vi "Audio ACQ & Store.vi"() -> ()   [LabVIEW 2020]
uses:
  support/typedefs/Record_States.ctl
  <vilib>/sound2/lvsound2.llb/Sound Input Task ID.ctl
  <vilib>/event_ctls.llb/usereventprio.ctl
  <vilib>/sound2/lvsound2.llb/Sampling Mode.ctl
  support/typedefs/Audio_Data.ctl
  <vilib>/sound2/lvsound2.llb/Sound Data Format.ctl
  <vilib>/sound2/lvsound2.llb/Sound Input Read (DBL).vi
panel:
  out "Audio":waveform(dbl)[](graph)
  in  "Refresh List":bool
  in  "Plot Selection":T1(array[cluster])
  in  "Audio Settings":T2={"Microphone Input Device"=0, "Channels"=1, "Audio Depth"=1, "Sampling Frequncy Hz"=44100.0} {"Sampling Frequncy Hz" items=["11025"=11025.0, "22050"=22050.0, "44100"=44100.0]; "Audio Depth" items=["8", "16"]; "Channels" items=["1", "2"]; "Microphone Input Device" items=["Microphone (USB 2.0 Camera)", "Microphone (2- High Definition Audio Device)", "Microphone (2- High Definition Audio Device)"]}
  in  "Clear":bool
  in  "Pause/Resume":bool
  in  "Stop":bool
  in  "Save":bool
  in  "Record":bool
  in  "Storage Path":path
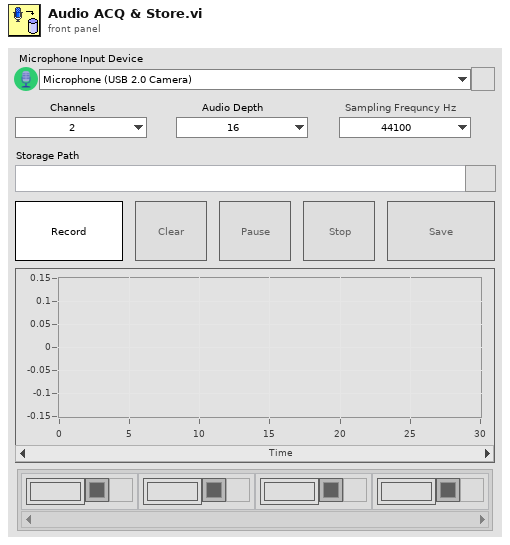
[diagram p1: front panel]
types:
  T1 = cluster{"Plot Name":string, "Plot Color":u32, "Visibility":bool}[]
  T2 = cluster{"Microphone Input Device":u32, "Channels":i32, "Audio Depth":i32, "Sampling Frequncy Hz":dbl}
  T3 = typedef "Record_States.ctl" = enum16{"Initialize", "Load Device List", "Load Device Info", "Respond UI", "Record", "Start ACQ", "Update Plot Propts", "Select Plots", "Clear", "Pause", "Resume", "Stop", "Save", "Exit"}
  T4 = typedef "Sound Input Task ID.ctl" = u32
  T5 = cluster{"channels":i32[], "depths":i32[], "minFreq":dbl, "maxFreq":dbl}[]
  T6 = enum8{"Enabled", "Disabled", "Disabled and Grayed Out"}
  T7 = cluster{"channels":i32[], "depths":i32[], "minFreq":dbl, "maxFreq":dbl}
  T8 = typedef "Audio_Data.ctl" = cluster{"Device":u32, "sound format":T9, "data":refnum<user-event>, "Pause?":bool}
  T9 = typedef "Sound Data Format.ctl" = cluster{"sample rate (S/s)":dbl, "number of channels":i32, "bits per sample":i32}
  T10 = typedef "usereventprio.ctl" = enum32{"high priority", "normal priority"}
  T11 = typedef "Sampling Mode.ctl" = i32
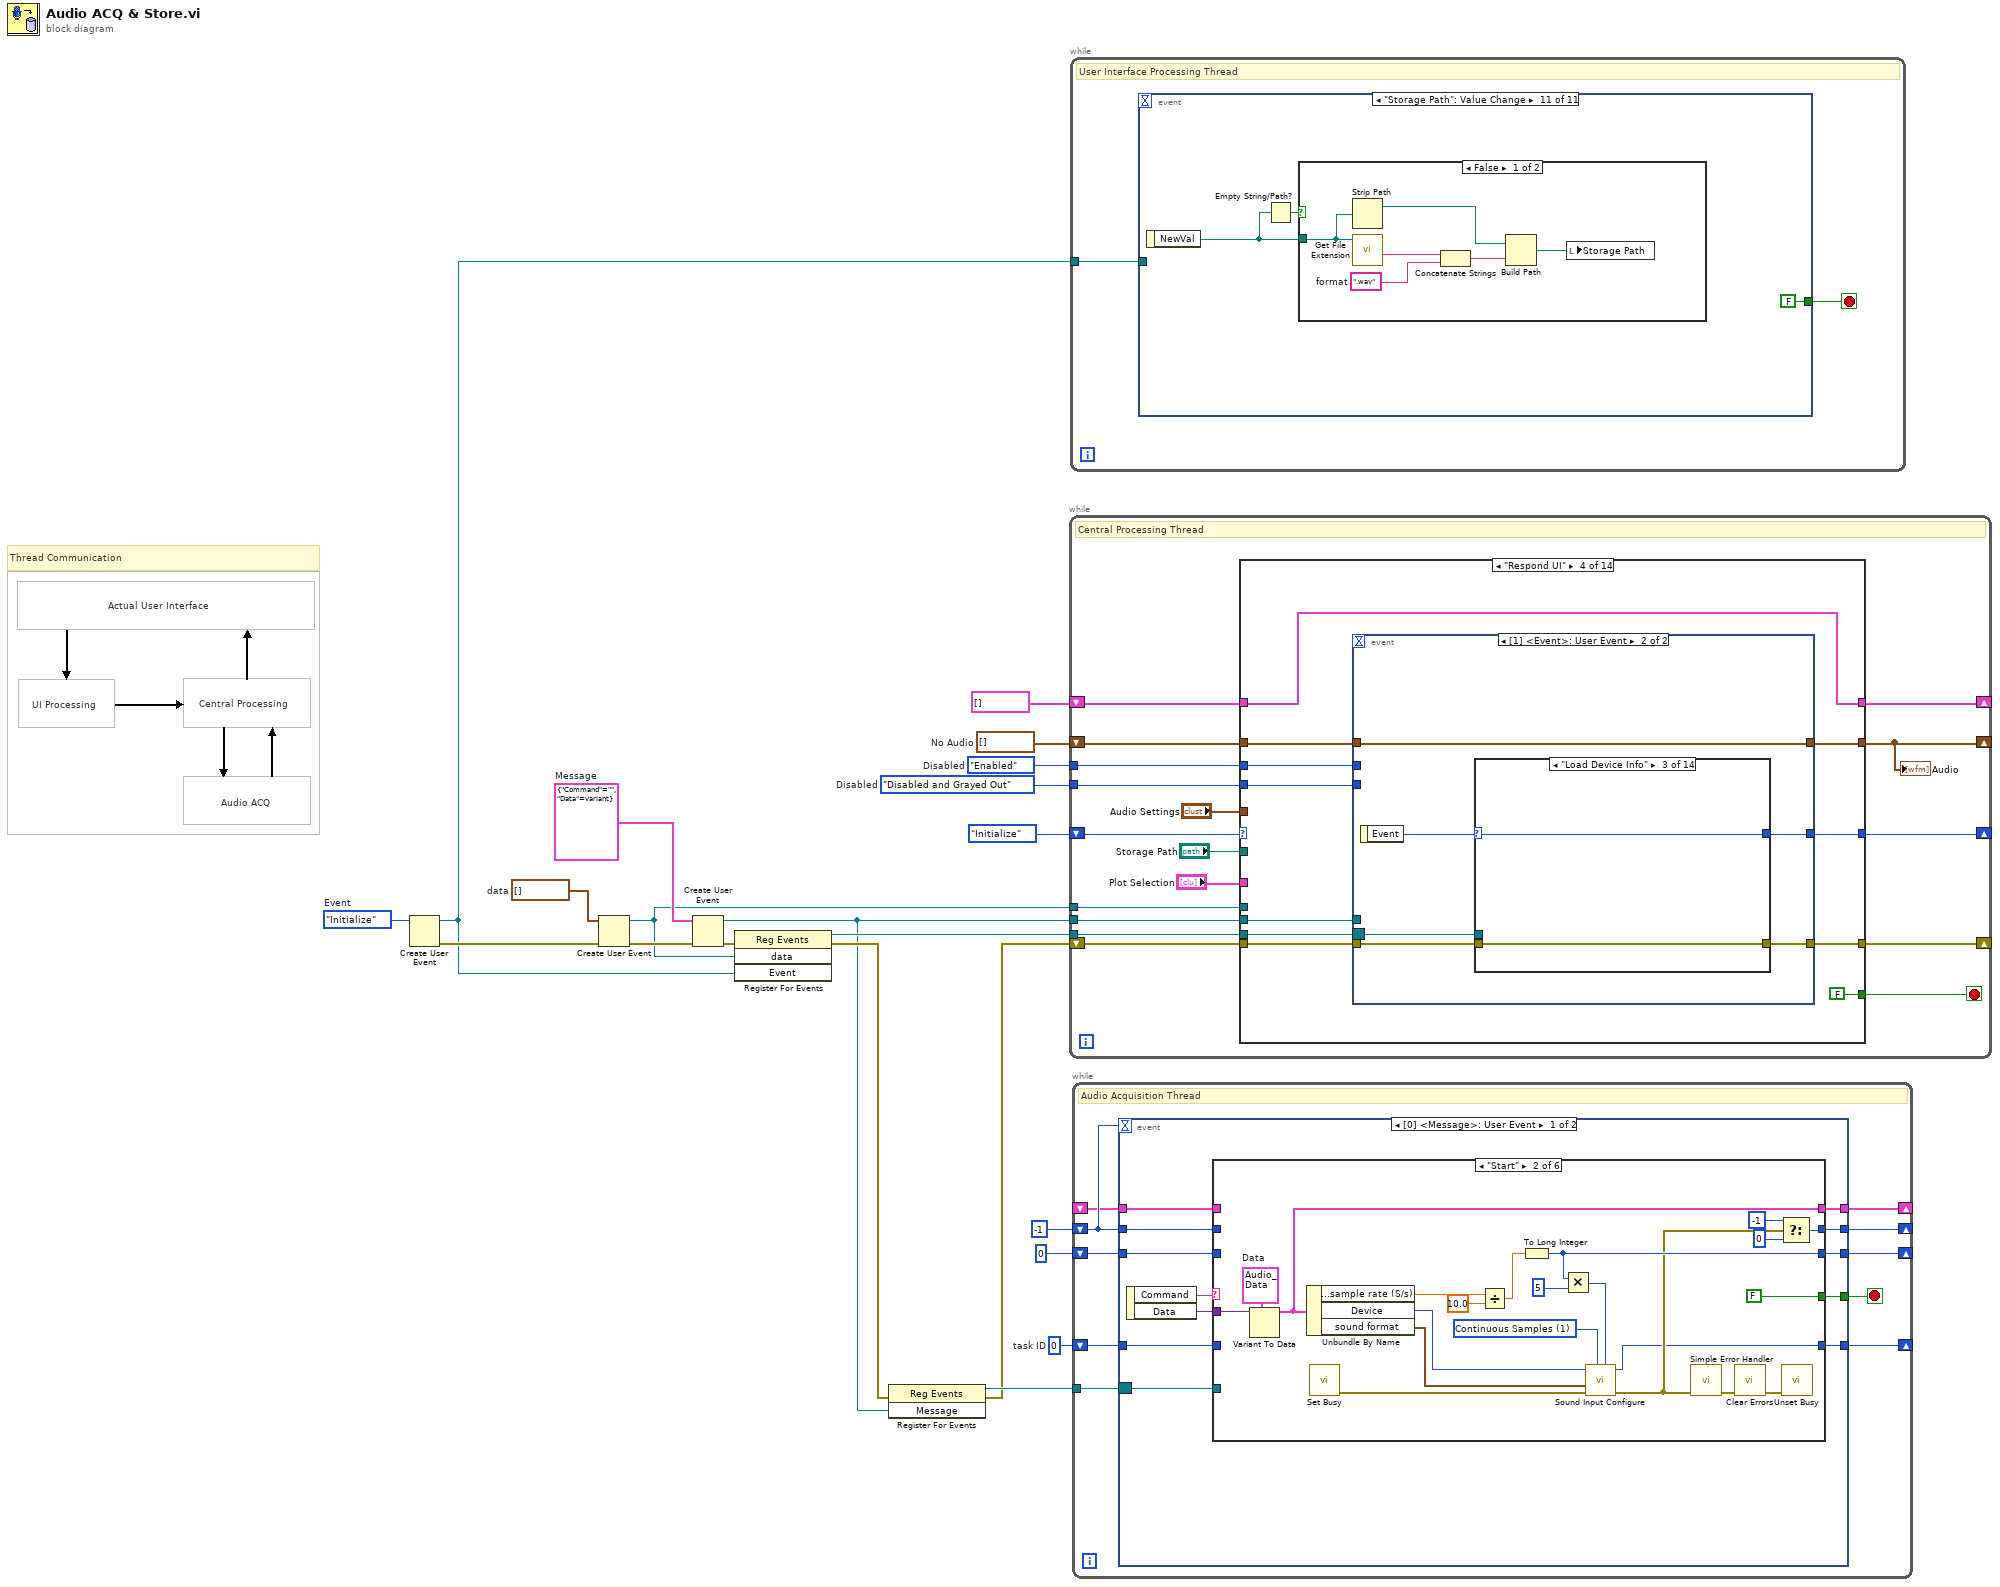
[diagram p0: block diagram]
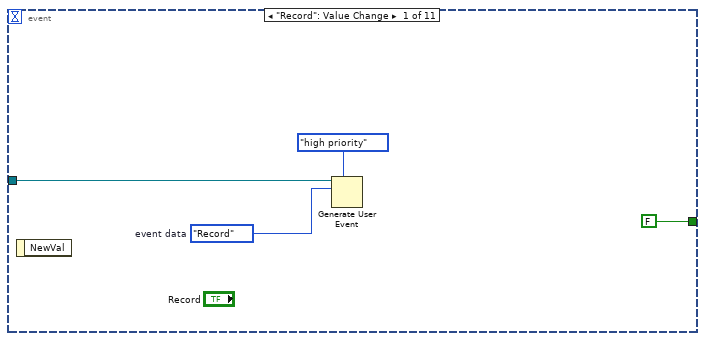
[diagram p2: hidden frame]
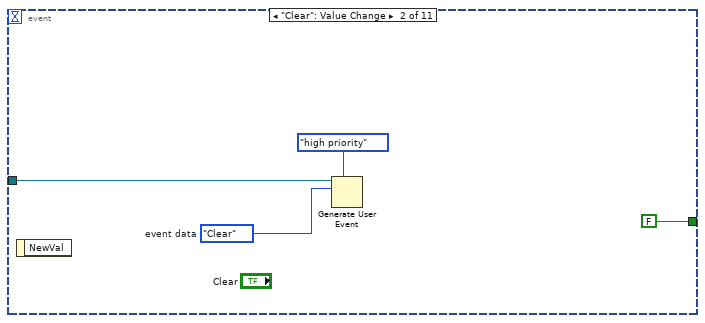
[diagram p3: hidden frame]
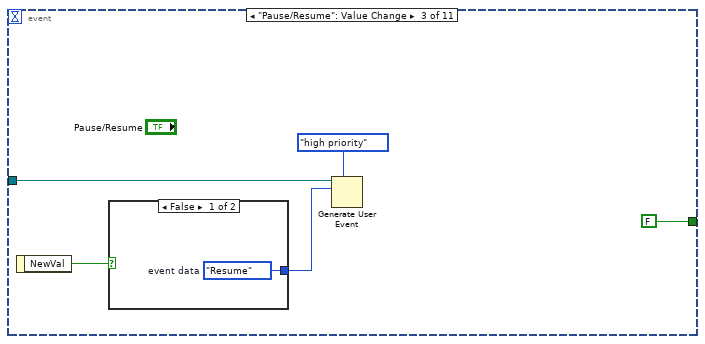
[diagram p4: hidden frame]
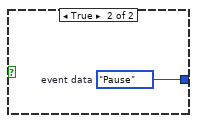
[diagram p5: hidden frame]
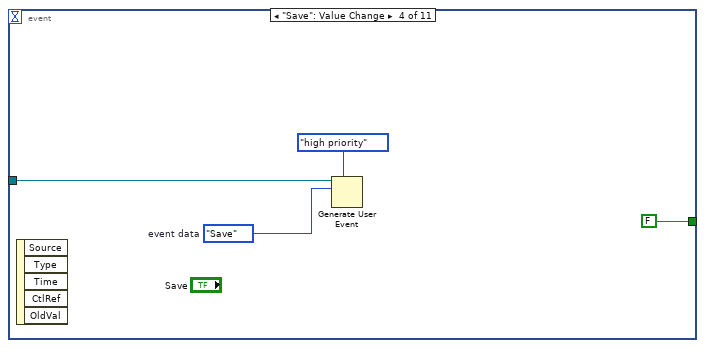
[diagram p6: hidden frame]
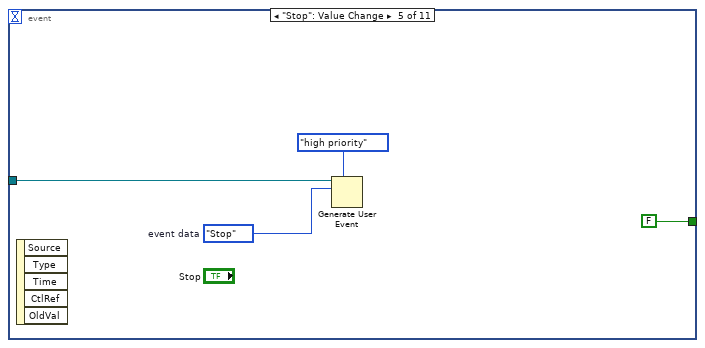
[diagram p7: hidden frame]
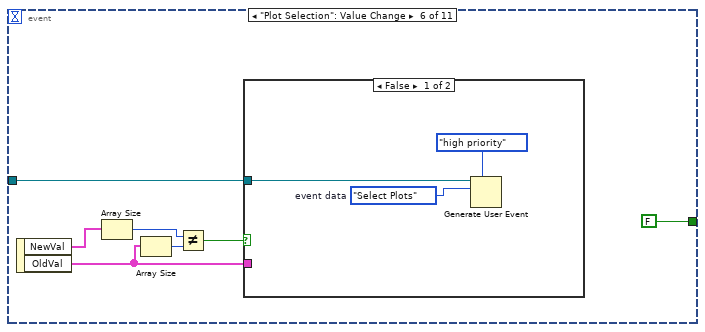
[diagram p8: hidden frame]
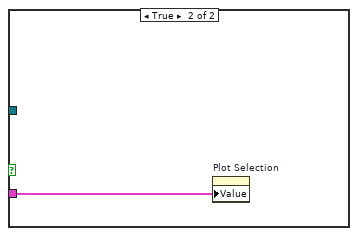
[diagram p9: hidden frame]
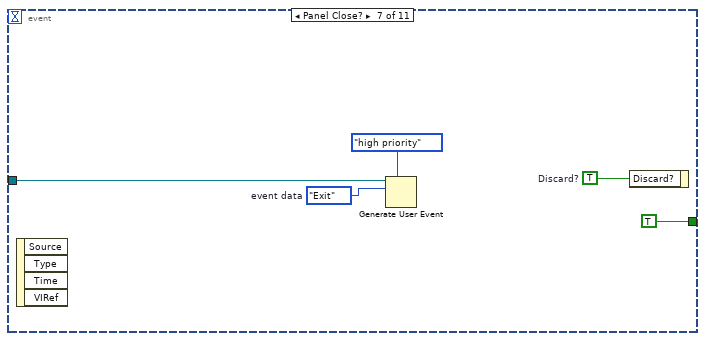
[diagram p10: hidden frame]
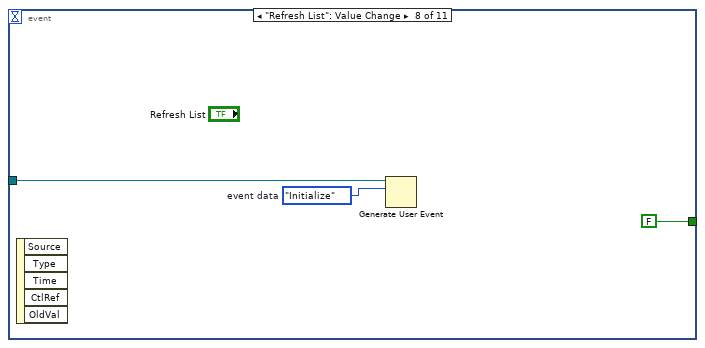
[diagram p11: hidden frame]
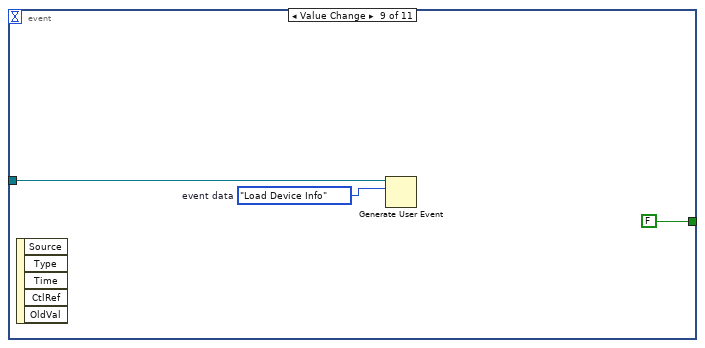
[diagram p12: hidden frame]
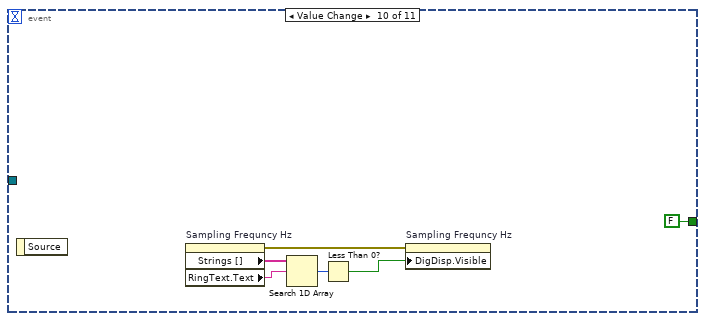
[diagram p13: hidden frame]
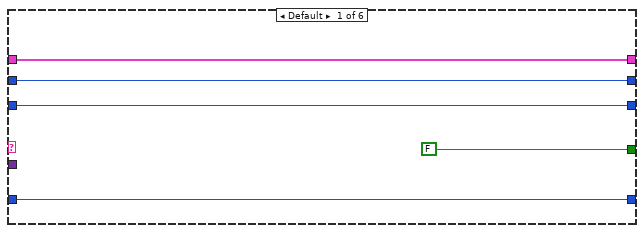
[diagram p15: hidden frame]
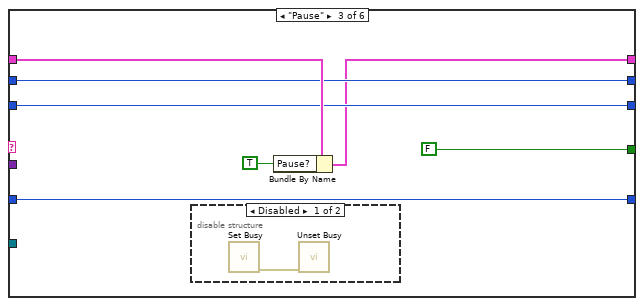
[diagram p16: hidden frame]
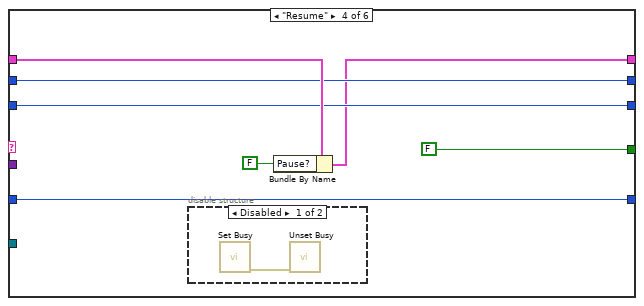
[diagram p18: hidden frame]
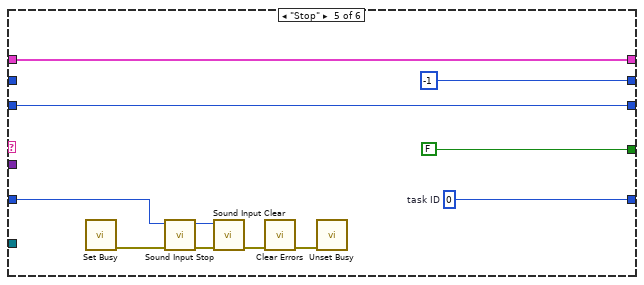
[diagram p20: hidden frame]
diagram:
  w5 = Record_States."Initialize"  # Event
  w8 = waveform(dbl)[] []  # No Audio
  w12 = waveform(dbl)[] []  # data
  w15 = T4 0  # task ID
  w19 = T6."Enabled"  # Disabled
  w18 = T6."Disabled and Grayed Out"  # Disabled
  w21 = cluster{"Command":string, "Data":variant} {"Command"="", "Data"=variant}  # Message
  # "Thread Communication"
  # "Actual User Interface"
  # "Audio ACQ"
  # "Central Processing"
  # "UI Processing"
  n1 = Create User Event(user event datatype=w5) -> (user event=w6:refnum<user-event>, error out=w7:errorcluster)  [unwired: 1 in]
  n2 = Create User Event(user event datatype=w12, error in=w7) -> (user event=w9:refnum<user-event>, error out=w13:errorcluster)
  n3 = Create User Event(user event datatype=w21, error in=w13) -> (user event=w1:refnum<user-event>, error out=w4:errorcluster)
  n4 = register-events(error in=w4, w9, w6) -> (reference out=w10:refnum<event-registration>, error out=w3:errorcluster)  [unwired: 1 in]
  n5 = register-events(error in=w3, w1) -> (reference out=w11:refnum<event-registration>, error out=w2:errorcluster)  [unwired: 1 in]
  n6 = while {
    tunnel: w1 -> [w29]
    shift-right: [w36] -> _
    shift-left: Record_States."Initialize" -> [w38]
    shift-right: [w35] -> _
    shift-left: w2 -> [w34]
    tunnel: w19 -> [w33]
    tunnel: w18 -> [w32]
    shift-right: [w31] -> _
    shift-left: T5 [] -> [w30]
    tunnel: w10 -> [w28]
    tunnel: w9 -> [w27]
    shift-right: [w23] -> _
    shift-left: w8 -> [w26]
    stop <- w37 stop-if-true
    # "Central Processing Thread"
    n7 = case shown="\"Respond UI\"" w38 {
      tunnel: [FALSE FALSE FALSE FALSE FALSE FALSE FALSE FALSE FALSE FALSE FALSE FALSE FALSE TRUE] -> w37
      tunnel: [Record_States."Load Device List" Record_States."Load Device Info" Record_States."Respond UI" w97 Record_States."Start ACQ" Record_States."Update Plot Propts" Record_States."Select Plots" Record_States."Respond UI" Record_States."Respond UI" Record_States."Respond UI" Record_States."Respond UI" Record_States."Respond UI" Record_States."Respond UI" Record_States."Respond UI"] -> w36
      tunnel: [w47 w59 w81 w96 w160 w172 w180 w191 w211 w235 w247 w264 w284 w307] -> w35
      tunnel: w34 -> [w46 w61 w83 w95 w164 w179 w184 w192 w216 w240 w252 w270 w288 w314]
      tunnel: w33 -> [w48 _ _ w93 w152 _ _ _ w205 w229 _ w258 _ _]
      tunnel: w32 -> [w42 _ _ w92 w146 _ _ _ w208 _ w241 w257 _ _]
      tunnel: [w54 w63 w80 w94 w163 w170 w183 w196 w215 w239 w251 w269 w281 w313] -> w31
      tunnel: w30 -> [w54 _ w80 w94 w163 w170 w183 w196 w215 w239 w251 w269 w281 w313]
      tunnel: w29 -> [_ _ _ w91 _ w171 _ _ _ w234 w246 w263 _ w300]
      tunnel: w28 -> [_ _ _ w90 _ _ _ _ _ _ _ _ _ _]
      tunnel: w27 -> [_ _ _ _ _ w168 _ _ _ _ _ _ _ _]
      tunnel: [w50 w62 w85 w88 w157 w167 w189 w195 w212 w232 w244 w254 w282 w302] -> w23
      tunnel: w26 -> [w50 w62 w85 w89 w157 w167 w189 w195 _ w232 w244 w254 w282 _]
      tunnel: "Audio Settings" -> [_ _ w84 _ _ w166 w182 _ _ _ _ _ w280 _]
      tunnel: "Storage Path" -> [_ _ _ _ _ _ _ _ _ _ _ _ w278 _]
      tunnel: "Plot Selection" -> [_ _ _ _ _ _ _ w190 _ _ _ _ _ _]
      frame "Initialize", Default {
        n8 = invoke on="Plot Selection" class="Arr (strict)" method="Reinit To Default"(error in=w46) -> (error out=w41:errorcluster)  [unwired: 2 in, 2 out]
        n9 = property on="Clear" class="Bool"(error in=w46, "DisabledEnum"=w42) -> (error out=w53:errorcluster)  [unwired: 1 in, 1 out]
        n10 = property on="Pause/Resume" class="Bool (strict)"(error in=w53, "DisabledEnum"=w42) -> (error out=w52:errorcluster)  [unwired: 1 in, 1 out]
        n11 = property on="Stop" class="Bool"(error in=w52, "DisabledEnum"=w42) -> (error out=w51:errorcluster)  [unwired: 1 in, 1 out]
        n12 = property on="Refresh List" class="Bool"(error in=w41, "Visible"=TRUE) -> (error out=w40:errorcluster)  [unwired: 1 in, 1 out]
        n13 = property on="Save" class="Bool"(error in=w51, "DisabledEnum"=w42) -> (error out=w44:errorcluster)  [unwired: 1 in, 1 out]
        n14 = property on="Plot Selection" class="Arr (strict)"(error in=w44, "DisabledEnum"=w42) -> (error out=w43:errorcluster)  [unwired: 1 in, 1 out]
        n15 = property on="Record" class="Bool"(error in=w43, "DisabledEnum"=w48) -> (error out=w49:errorcluster)  [unwired: 1 in, 1 out]
        n16 = property on="Audio Settings" class="Clust (strict)"(error in=w49, "DisabledEnum"=w48) -> (error out=w45:errorcluster)  [unwired: 1 in, 1 out]
        n17 = Merge Errors(w45, w40) -> (w47:errorcluster)
      }
      frame "Load Device List" {
        w58 = TRUE  # isInput?
        n18 = call <vilib>:"Get Num Devices.vi"("error in (no error)"=w61) -> ("error out"=w59:errorcluster, "Number of Input Devices"=w60:i32)  [unwired: 8 in, 1 out]
        n19 = for {
          N: w60 -> [_]
          tunnel: [w67] -> w64 mode=indexing if=w72
          tunnel: [w68] -> w63 mode=indexing if=w72
          tunnel: w58 -> [w70]
          i -> [w71]
          n20 = call <vilib>:"Sound Device Info.vi"("device"=w71, "isInput?"=w70) -> ("Device Name"=w67:string, "Capabilities"=w68:T7, "error out"=w69:errorcluster)  [unwired: 11 in]
          n21 = Unbundle By Name(w69) -> ("status"=w73:bool)
          n22 = Not(x=w73) -> (.not. x?=w72:bool)
        }
        n23 = property on="Microphone Input Device" class="Ring (strict)"("Strings []"=w64, "Value"=u32 0) -> ()  [unwired: 2 in, 2 out]
      }
      frame "Load Device Info" {
        n24 = Unbundle By Name(w84) -> ("Microphone Input Device"=w79:u32)
        n25 = Index Array(array=w80, index=w79) -> (element=w78:T7)
        n26 = Unbundle By Name(w78) -> ("channels"=w76:i32[], "depths"=w77:i32[])
        n27 = Number To Decimal String(number=w76) -> (decimal integer string=w75:string[])  [unwired: 1 in]
        n28 = Number To Decimal String(number=w77) -> (decimal integer string=w74:string[])  [unwired: 1 in]
        n29 = property on="Audio Depth" class="Ring (strict)"(error in=w83, "Strings []"=w74) -> (error out=w82:errorcluster)  [unwired: 1 in, 1 out]
        n30 = property on="Channels" class="Ring (strict)"(error in=w82, "Strings []"=w75) -> (error out=w81:errorcluster)  [unwired: 1 in, 1 out]
      }
      frame "Respond UI" {
        n31 = event shown="[1] <Event>: User Event" {
          selector: w90 -> [_ w105]
          dyn-events: _ -> [_ _]
          timeout: _ -> [_ _]
          tunnel: [Record_States."Respond UI" w109] -> w97
          tunnel: [w102 w106] -> w96
          tunnel: w95 -> [w102 w107]
          tunnel: w93 -> [_ _]
          tunnel: w92 -> [_ _]
          tunnel: w91 -> [_ _]
          tunnel: w89 -> [w100 w108]
          tunnel: [w99 w108] -> w88
          event User Event {
            n32 = event-data() -> ("data"=w101:waveform(dbl)[])  [unwired: 1 in]
            n33 = call "append_audio.vi"("latest"=w101, "Old"=w100) -> ("Appended"=w99:waveform(dbl)[])  [unwired: 4 in]
          }
          event User Event {
            n34 = event-data() -> ("Event"=w104:T3)  [unwired: 1 in]
            n35 = case shown="\"Load Device Info\"" w104 {
              selector: w104 -> [w110 w112 w114 w116 w118 w120 w122 w124 w128 w132 w134 w136 w140 w142]
              tunnel: [w110 w112 w114 w116 w118 w120 w122 w124 w128 w132 w134 w136 w140 w142] -> w109
              tunnel: w107 -> [w111 w113 w115 w117 w119 w121 w123 w125 w129 w133 w135 w137 w141 w145]
              tunnel: [w111 w113 w115 w117 w119 w121 w123 w125 w127 w131 w135 w137 w139 w144] -> w106
              tunnel: w105 -> [_ _ _ _ _ _ _ _ w126 w130 _ _ w138 w143]
              frame "Initialize" {
              }
              frame "Load Device List" {
              }
              frame "Load Device Info" {
              }
              frame "Respond UI" {
              }
              frame "Record" {
              }
              frame "Start ACQ" {
              }
              frame "Update Plot Propts" {
              }
              frame "Select Plots" {
              }
              frame "Clear" {
                n36 = Flush Event Queue(0:w126, 3:w129) -> (11:w127:errorcluster)  [unwired: 4 in, 2 out]
              }
              frame "Pause" {
                n37 = Flush Event Queue(0:w130, 3:w133) -> (11:w131:errorcluster)  [unwired: 4 in, 2 out]
              }
              frame "Resume" {
              }
              frame "Save" {
              }
              frame "Exit" {
                n38 = Flush Event Queue(0:w138, 3:w141) -> (11:w139:errorcluster)  [unwired: 4 in, 2 out]
              }
              frame "Stop" {
                n39 = Flush Event Queue(0:w143, 3:w145) -> (11:w144:errorcluster)  [unwired: 4 in, 2 out]
              }
            }
          }
        }
      }
      frame "Record" {
        n40 = call <vilib>:"Set Busy.vi"("error in (no error)"=w164) -> ("error out"=w148:errorcluster)  [unwired: 9 in, 1 out]
        n41 = property on="Record" class="Bool"(error in=w148, "DisabledEnum"=w146) -> (error out=w156:errorcluster)  [unwired: 1 in, 1 out]
        n42 = property on="Save" class="Bool"(error in=w148, "DisabledEnum"=w146) -> (error out=w147:errorcluster)  [unwired: 1 in, 1 out]
        n43 = property on="Audio Settings" class="Clust (strict)"(error in=w156, "DisabledEnum"=w146) -> (error out=w155:errorcluster)  [unwired: 1 in, 1 out]
        n44 = property on="Clear" class="Bool"(error in=w155, "DisabledEnum"=w152) -> (error out=w159:errorcluster)  [unwired: 1 in, 1 out]
        n45 = property on="Refresh List" class="Bool"(error in=w147, "Visible"=FALSE) -> (error out=w149:errorcluster)  [unwired: 1 in, 1 out]
        n46 = property on="Pause/Resume" class="Bool (strict)"(error in=w159, "DisabledEnum"=w152) -> (error out=w158:errorcluster)  [unwired: 1 in, 1 out]
        n47 = property on="Stop" class="Bool"(error in=w158, "DisabledEnum"=w152) -> (error out=w154:errorcluster)  [unwired: 1 in, 1 out]
        n48 = property on="Plot Selection" class="Arr (strict)"(error in=w154, "DisabledEnum"=w152) -> (error out=w153:errorcluster)  [unwired: 1 in, 1 out]
        n49 = Merge Errors(w153, w149) -> (w150:errorcluster)
        n50 = call <vilib>:"Unset Busy.vi"("error in (no error)"=w150) -> ("error out"=w160:errorcluster)  [unwired: 10 in]
      }
      frame "Start ACQ" {
        w175 = cluster{"Command":string, "Data":variant} {"Command"="Start", "Data"=variant}  # start
        n51 = call <vilib>:"Set Busy.vi"("error in (no error)"=w179) -> ("error out"=w173:errorcluster)  [unwired: 9 in, 1 out]
        n52 = call "Build_ACQ_cfg.vi"("User Event in"=w168, "Audio Settings"=w166, "Audio Device Details"=w170) -> ("Audio DAQ cfg"=w169:T8)
        n53 = To Variant(anything=w169) -> (Variant=w165:variant)
        n54 = Bundle By Name(cluster=w175, "Data"=w165) -> (w174:cluster{"Command":string, "Data":variant})
        n55 = Generate User Event(user event=w171, event data cluster=w174, error in=w173) -> (error out=w176:errorcluster)  [unwired: 1 in, 1 out]
        n56 = call <vilib>:"Unset Busy.vi"("error in (no error)"=w176) -> ("error out"=w172:errorcluster)  [unwired: 10 in]
      }
      frame "Update Plot Propts" {
        n57 = call <vilib>:"Set Busy.vi"("error in (no error)"=w184) -> ("error out"=w181:errorcluster)  [unwired: 9 in, 1 out]
        n58 = call "Build_Plot_Selection-Acquire.vi"("Audio Device Details"=w183, "Audio Settings"=w182, "error in (no error)"=w181) -> ("error out"=w185:errorcluster, "Plot Selection"=w186:T1)  [unwired: 7 in]
        n59 = local write "Plot Selection"(w186) -> ()
        n60 = call <vilib>:"Unset Busy.vi"("error in (no error)"=w185) -> ("error out"=w180:errorcluster)  [unwired: 10 in]
      }
      frame "Select Plots" {
        n61 = for {
          shift-right: [w204] -> w191
          shift-left: w192 -> [w198]
          tunnel: w190 -> [w203] mode=indexing
          i -> [w197]
          n62 = Unbundle By Name(w203) -> ("Plot Name"=w202:string, "Plot Color"=w201:u32, "Visibility"=w200:bool)
          n63 = property on="Audio" class="WFGraph (strict)"(error in=w198, "Active Plot"=w197) -> (error out=w199:errorcluster)  [unwired: 1 in, 1 out]
          n64 = property on="Audio" class="WFGraph (strict)"(error in=w199, "Plot.Plot Name"=w202, "Plot.Plot Color"=w201, "Plot.Visible?"=w200) -> (error out=w204:errorcluster)  [unwired: 1 in, 1 out]
        }
      }
      frame "Clear" {
        w212 = waveform(dbl)[] []  # No Audio
        n65 = call <vilib>:"Set Busy.vi"("error in (no error)"=w216) -> ("error out"=w210:errorcluster)  [unwired: 9 in, 1 out]
        n66 = property on="Stop" class="Bool"(error in=w210) -> (error out=w207:errorcluster, "DisabledEnum"=w209:T6)  [unwired: 1 in, 1 out]
        n67 = case shown="Default" w209 {
          tunnel: w208 -> [w217 w221]
          tunnel: w207 -> [w219 w228]
          tunnel: [w218 w226] -> w206
          tunnel: w205 -> [_ w224]
          frame "Enabled" {
            # "Audio Not Stopped"
            n68 = property on="Save" class="Bool"(error in=w219, "DisabledEnum"=w217) -> (error out=w218:errorcluster)  [unwired: 1 in, 1 out]
          }
          frame Default {
            # "Audio Stopped"
            n69 = property on="Clear" class="Bool"(error in=w228, "DisabledEnum"=w221) -> (error out=w227:errorcluster)  [unwired: 1 in, 1 out]
            n70 = property on="Save" class="Bool"(error in=w227, "DisabledEnum"=w221) -> (error out=w223:errorcluster)  [unwired: 1 in, 1 out]
            n71 = property on="Refresh List" class="Bool"("Visible"=TRUE) -> ()  [unwired: 2 in, 2 out]
            n72 = property on="Plot Selection" class="Arr (strict)"(error in=w223, "DisabledEnum"=w221) -> (error out=w222:errorcluster)  [unwired: 1 in, 1 out]
            n73 = property on="Audio Settings" class="Clust (strict)"(error in=w222, "DisabledEnum"=w224) -> (error out=w225:errorcluster)  [unwired: 1 in, 1 out]
            n74 = property on="Record" class="Bool"(error in=w225, "DisabledEnum"=w224) -> (error out=w226:errorcluster)  [unwired: 1 in, 1 out]
          }
        }
        n75 = call <vilib>:"Unset Busy.vi"("error in (no error)"=w206) -> ("error out"=w211:errorcluster)  [unwired: 10 in]
      }
      frame "Pause" {
        w233 = cluster{"Command":string, "Data":variant} {"Command"="Pause", "Data"=variant}  # Pause
        n76 = call <vilib>:"Set Busy.vi"("error in (no error)"=w240) -> ("error out"=w231:errorcluster)  [unwired: 9 in, 1 out]
        n77 = property on="Save" class="Bool"(error in=w231, "DisabledEnum"=w229) -> (error out=w230:errorcluster)  [unwired: 1 in, 1 out]
        n78 = Generate User Event(user event=w234, event data cluster=w233, error in=w230) -> (error out=w236:errorcluster)  [unwired: 1 in, 1 out]
        n79 = call <vilib>:"Unset Busy.vi"("error in (no error)"=w236) -> ("error out"=w235:errorcluster)  [unwired: 10 in]
      }
      frame "Resume" {
        w245 = cluster{"Command":string, "Data":variant} {"Command"="Resume", "Data"=variant}  # Resume
        n80 = call <vilib>:"Set Busy.vi"("error in (no error)"=w252) -> ("error out"=w243:errorcluster)  [unwired: 9 in, 1 out]
        n81 = property on="Save" class="Bool"(error in=w243, "DisabledEnum"=w241) -> (error out=w242:errorcluster)  [unwired: 1 in, 1 out]
        n82 = Generate User Event(user event=w246, event data cluster=w245, error in=w242) -> (error out=w248:errorcluster)  [unwired: 1 in, 1 out]
        n83 = call <vilib>:"Unset Busy.vi"("error in (no error)"=w248) -> ("error out"=w247:errorcluster)  [unwired: 10 in]
      }
      frame "Stop" {
        w265 = cluster{"Command":string, "Data":variant} {"Command"="Stop", "Data"=variant}  # Stop
        n84 = call <vilib>:"Set Busy.vi"("error in (no error)"=w270) -> ("error out"=w261:errorcluster)  [unwired: 9 in, 1 out]
        n85 = property on="Pause/Resume" class="Bool (strict)"(error in=w261, "DisabledEnum"=w257, "Value"=FALSE) -> (error out=w253:errorcluster)  [unwired: 1 in, 1 out]
        n86 = property on="Stop" class="Bool"(error in=w253, "DisabledEnum"=w257) -> (error out=w260:errorcluster)  [unwired: 1 in, 1 out]
        n87 = property on="Record" class="Bool"(error in=w260, "DisabledEnum"=w258) -> (error out=w262:errorcluster)  [unwired: 1 in, 1 out]
        n88 = Empty Array?(array=w254) -> (empty?=w255:bool)
        n89 = case shown="False" w255 {
          tunnel: w262 -> [w273 w274]
          tunnel: [w272 w274] -> w259
          tunnel: w258 -> [w271 _]
          frame False {
            n90 = property on="Save" class="Bool"(error in=w273, "DisabledEnum"=w271) -> (error out=w272:errorcluster)  [unwired: 1 in, 1 out]
          }
          frame True {
          }
        }
        n91 = Generate User Event(user event=w263, event data cluster=w265, error in=w259) -> (error out=w266:errorcluster)  [unwired: 1 in, 1 out]
        n92 = call <vilib>:"Unset Busy.vi"("error in (no error)"=w266) -> ("error out"=w264:errorcluster)  [unwired: 10 in]
      }
      frame "Save" {
        n93 = call "Build_Device_Details.vi"("Audio Settings"=w280, "Audio Device Details"=w281) -> ("Depth"=w279:i32)  [unwired: 4 in, 5 out]
        n94 = call <vilib>:"Set Busy.vi"("error in (no error)"=w288) -> ("error out"=w285:errorcluster)  [unwired: 9 in, 1 out]
        n95 = Not A Number/Path/Refnum?(number/path/refnum=w278) -> (NaN/Path/Refnum?=w275:bool)
        n96 = Empty String/Path?(string/path=w278) -> (empty?=w276:bool)
        n97 = Or(x=w275, y=w276) -> (x .or. y?=w277:bool)
        n98 = case shown="False" w277 {
          tunnel: w285 -> [w295 w297]
          tunnel: [w290 w297] -> w283
          tunnel: w278 -> [w293 _]
          tunnel: w282 -> [w292 _]
          tunnel: w279 -> [w289 _]
          frame False {
            n99 = call <vilib>:"Sound File Write Simple.vi"("error in (no error)"=w295, "bits per sample"=w289, "data"=w292, "path"=w293) -> ("error out"=w294:errorcluster)  [unwired: 6 in, 1 out]
            n100 = call <vilib>:"Simple Error Handler.vi"("error in (no error)"=w294) -> ("error out"=w291:errorcluster)  [unwired: 4 in, 4 out]
            n101 = call <vilib>:"Clear Errors.vi"("error in (no error)"=w291) -> ("error out"=w290:errorcluster)  [unwired: 5 in, 1 out]
          }
          frame True {
            w296 = "Enter Valid Path"  # message
            n102 = One Button Dialog(message=w296) -> ()  [unwired: 1 in, 1 out]
          }
        }
        n103 = call <vilib>:"Unset Busy.vi"("error in (no error)"=w283) -> ("error out"=w284:errorcluster)  [unwired: 10 in]
      }
      frame "Exit" {
        w298 = cluster{"Command":string, "Data":variant} {"Command"="Stop", "Data"=variant}  # Stop
        w302 = waveform(dbl)[] []  # No Audio
        w309 = cluster{"Command":string, "Data":variant} {"Command"="Exit", "Data"=variant}  # Exit
        n104 = call <vilib>:"Set Busy.vi"("error in (no error)"=w314) -> ("error out"=w308:errorcluster)  [unwired: 9 in, 1 out]
        n105 = Generate User Event(user event=w300, event data cluster=w298, error in=w308) -> (user event out=w299:refnum<user-event>, error out=w301:errorcluster)  [unwired: 1 in]
        n106 = Generate User Event(user event=w299, event data cluster=w309, error in=w301) -> (user event out=w305:refnum<user-event>, error out=w310:errorcluster)  [unwired: 1 in]
        n107 = flat-sequence {
          tunnel: w305 -> [w316]
          tunnel: w310 -> [w317]
          tunnel: [w317] -> w304
          tunnel: [w316] -> w303
          tunnel: [w319] -> w306
          tunnel: w304 -> [w320]
          tunnel: w303 -> [w318]
          frame #0 {
            n108 = Wait (ms)(milliseconds to wait=u32 100) -> ()  [unwired: 1 out]
          }
          frame #1 {
            n109 = Destroy User Event(user event=w318, error in=w320) -> (error out=w319:errorcluster)
          }
        }
        n110 = call <vilib>:"Unset Busy.vi"("error in (no error)"=w306) -> ("error out"=w307:errorcluster)  [unwired: 10 in]
      }
    }
    "Audio" <- w23
  }
  n111 = while {
    tunnel: w6 -> [w322]
    stop <- w321 stop-if-true
    # "User Interface Processing Thread"
    n112 = event shown="[10] \"Storage Path\": Value Change" {
      selector: _ -> [_ _ _ _ _ _ _ _ _ _ _]
      dyn-events: _ -> [_ _ _ _ _ _ _ _ _ _ _]
      timeout: _ -> [_ _ _ _ _ _ _ _ _ _ _]
      tunnel: w322 -> [w326 w330 w335 w341 w345 w346 w360 w363 w366 _ _]
      tunnel: [FALSE FALSE FALSE FALSE FALSE FALSE TRUE FALSE FALSE FALSE FALSE] -> w321
      event "Record": Value Change {
        w323 = Record_States."Record"  # event data
        n113 = event-data() -> ()  [unwired: 1 in, 1 out]
        n114 = Generate User Event(priority (normal)=usereventprio."high priority", user event=w326, event data cluster=w323) -> ()  [unwired: 1 in, 2 out]
      }
      event "Clear": Value Change {
        w327 = Record_States."Clear"  # event data
        n115 = event-data() -> ()  [unwired: 1 in, 1 out]
        n116 = Generate User Event(priority (normal)=usereventprio."high priority", user event=w330, event data cluster=w327) -> ()  [unwired: 1 in, 2 out]
      }
      event "Pause/Resume": Value Change {
        n117 = event-data() -> ("NewVal"=w331:bool)  [unwired: 1 in]
        n118 = case shown="False" w331 {
          tunnel: [w336 w337] -> w332
          frame False {
            w336 = Record_States."Resume"  # event data
          }
          frame True {
            w337 = Record_States."Pause"  # event data
          }
        }
        n119 = Generate User Event(priority (normal)=usereventprio."high priority", user event=w335, event data cluster=w332) -> ()  [unwired: 1 in, 2 out]
      }
      event "Save": Value Change {
        w338 = Record_States."Save"  # event data
        n120 = event-data() -> ()  [unwired: 1 in, 5 out]
        n121 = Generate User Event(priority (normal)=usereventprio."high priority", user event=w341, event data cluster=w338) -> ()  [unwired: 1 in, 2 out]
      }
      event "Stop": Value Change {
        w342 = Record_States."Stop"  # event data
        n122 = event-data() -> ()  [unwired: 1 in, 5 out]
        n123 = Generate User Event(priority (normal)=usereventprio."high priority", user event=w345, event data cluster=w342) -> ()  [unwired: 1 in, 2 out]
      }
      event "Plot Selection": Value Change {
        n124 = event-data() -> ("NewVal"=w348:T1, "OldVal"=w347:T1)  [unwired: 1 in]
        n125 = Array Size(array=w348) -> (size(s)=w351:i32)
        n126 = Array Size(array=w347) -> (size(s)=w350:i32)
        n127 = Not Equal?(x=w351, y=w350) -> (x != y?=w349:bool)
        n128 = case shown="False" w349 {
          tunnel: w347 -> [_ w356]
          tunnel: w346 -> [w353 _]
          frame False {
            w355 = Record_States."Select Plots"  # event data
            n129 = Generate User Event(priority (normal)=usereventprio."high priority", user event=w353, event data cluster=w355) -> ()  [unwired: 1 in, 2 out]
          }
          frame True {
            n130 = property on="Plot Selection" class="Arr (strict)"("Value"=w356) -> ()  [unwired: 2 in, 2 out]
          }
        }
      }
      event Panel Close? {
        w357 = TRUE  # Discard?
        w359 = Record_States."Exit"  # event data
        n131 = event-data() -> ()  [unwired: 1 in, 4 out]
        n132 = Generate User Event(priority (normal)=usereventprio."high priority", user event=w360, event data cluster=w359) -> ()  [unwired: 1 in, 2 out]
        n133 = event-data("Discard?"=w357) -> ()  [unwired: 1 in, 1 out]
      }
      event "Refresh List": Value Change {
        w362 = Record_States."Initialize"  # event data
        n134 = event-data() -> ()  [unwired: 1 in, 5 out]
        n135 = Generate User Event(user event=w363, event data cluster=w362) -> ()  [unwired: 2 in, 2 out]
      }
      event "Audio Settings.Microphone Input Device": Value Change {
        w365 = Record_States."Load Device Info"  # event data
        n136 = event-data() -> ()  [unwired: 1 in, 5 out]
        n137 = Generate User Event(user event=w366, event data cluster=w365) -> ()  [unwired: 2 in, 2 out]
      }
      event "Audio Settings.Sampling Frequncy Hz": Value Change {
        n138 = event-data() -> ()  [unwired: 1 in, 1 out]
        n139 = property on="Sampling Frequncy Hz" class="Ring (strict)"() -> (error out=w370:errorcluster, "Strings []"=w372:string[], "RingText.Text"=w373:string)  [unwired: 2 in, 1 out]
        n140 = Search 1D Array(1D array=w372, element=w373) -> (index of element=w371:i32)  [unwired: 1 in]
        n141 = Less Than 0?(x=w371) -> (x < 0?=w369:bool)
        n142 = property on="Sampling Frequncy Hz" class="Ring (strict)"(error in=w370, "DigDisp.Visible"=w369) -> ()  [unwired: 1 in, 2 out]
      }
      event "Storage Path": Value Change {
        n143 = event-data() -> ("NewVal"=w375:path)  [unwired: 1 in]
        n144 = Empty String/Path?(string/path=w375) -> (empty?=w374:bool)
        n145 = case shown="False" w374 {
          tunnel: w375 -> [w377 _]
          frame False {
            w381 = ".wav"  # format
            n146 = Strip Path(path=w377) -> (stripped path=w378:path)  [unwired: 1 out]
            n147 = call <vilib>:"Get File Extension.vi"("file"=w377) -> ("filename without extension"=w382:string)  [unwired: 6 in, 4 out]
            n148 = Concatenate Strings(w382, w381) -> (w380:string)
            n149 = Build Path(base path=w378, name or relative path=w380) -> (appended path=w379:path)
            n150 = local write "Storage Path"(w379) -> ()
          }
          frame True {
          }
        }
      }
    }
  }
  n151 = while {
    tunnel: w11 -> [w392]
    shift-right: [w390] -> _
    shift-left: -1 -> [w389]
    shift-right: [w388] -> _
    shift-left: w15 -> [w387]
    shift-right: [w386] -> _
    shift-left: 0 -> [w385]
    shift-right: [w384] -> _
    shift-left: _ -> [w383]
    stop <- w391 stop-if-true
    # "Audio Acquisition Thread"
    n152 = event shown="[0] <Message>: User Event" {
      selector: w392 -> [w393 _]
      dyn-events: _ -> [_ _]
      timeout: w389 -> [_ _]
      tunnel: [w403 FALSE] -> w391
      tunnel: [w401 w474] -> w390
      tunnel: w389 -> [w402 w479]
      tunnel: [w399 w477] -> w388
      tunnel: w387 -> [w398 w478]
      tunnel: [w397 w476] -> w386
      tunnel: w385 -> [w396 w476]
      tunnel: [w395 w472] -> w384
      tunnel: w383 -> [w394 w472]
      event User Event {
        n153 = event-data() -> ("Command"=w404:string, "Data"=w400:variant)  [unwired: 1 in]
        n154 = case shown="\"Start\"" w404 {
          tunnel: [FALSE FALSE FALSE FALSE FALSE TRUE] -> w403
          tunnel: w402 -> [w405 _ w433 w441 _ w465]
          tunnel: [w405 w422 w433 w441 -1 w465] -> w401
          tunnel: w400 -> [_ w428 _ _ _ _]
          tunnel: [w406 w410 w434 w442 w453 w464] -> w399
          tunnel: w398 -> [w406 _ w434 w442 w452 w464]
          tunnel: [w407 w412 w435 w443 w454 w463] -> w397
          tunnel: w396 -> [w407 _ w435 w443 w454 w463]
          tunnel: [w408 w424 w432 w440 w455 w462] -> w395
          tunnel: w394 -> [w408 _ w436 w444 w455 w462]
          tunnel: w393 -> [_ _ _ _ _ w458]
          frame Default {
          }
          frame "Start" {
            w427 = T8 {"Device"=0, "sound format"={"sample rate (S/s)"=22050.0, "number of channels"=2, "bits per sample"=16}, "data"=refnum, "Pause?"=FALSE}  # Data
            w429 = T11 1 items=["Finite Samples", "Continuous Samples"] ("sample mode")
            n155 = Variant To Data(type=w427, Variant=w428) -> (data=w424:T8)  [unwired: 1 in, 1 out]
            n156 = Unbundle By Name(w424) -> ("sound format.sample rate (S/s)"=w415:dbl, "Device"=w426:u32, "sound format"=w425:T9)
            n157 = call <vilib>:"Set Busy.vi"() -> ("error out"=w418:errorcluster)  [unwired: 10 in, 1 out]
            n158 = Divide(x=w415, y=10.0) -> (x/y=w413:dbl)
            n159 = To Long Integer(number=w413) -> (32bit integer=w412:i32)
            n160 = Multiply(x=w412, y=5) -> (x*y=w420:i32)
            n161 = call <vilib>:"Sound Input Configure.vi"("number of samples/ch"=w420, "sample mode"=w429, "error in (no error)"=w418, "sound format"=w425, "device ID"=w426) -> ("error out"=w411:errorcluster, "task ID"=w410:T4)  [unwired: 5 in]
            n162 = call <vilib>:"Simple Error Handler.vi"("error in (no error)"=w411) -> ("error out"=w417:errorcluster)  [unwired: 4 in, 4 out]
            n163 = call <vilib>:"Clear Errors.vi"("error in (no error)"=w417) -> ("error out"=w416:errorcluster)  [unwired: 5 in, 1 out]
            n164 = Select(t=-1, s=w411, f=0) -> (s? t:f=w422:i32)
            n165 = call <vilib>:"Unset Busy.vi"("error in (no error)"=w416) -> ()  [unwired: 10 in, 1 out]
          }
          frame "Pause" {
            n166 = disable-structure shown="Disabled" {
              frame Disabled {
                n167 = call <vilib>:"Set Busy.vi"() -> ("error out"=w438:errorcluster)  [unwired: 10 in, 1 out]
                n168 = call <vilib>:"Unset Busy.vi"("error in (no error)"=w438) -> ()  [unwired: 10 in, 1 out]
              }
              frame Enabled {
              }
            }
            n169 = Bundle By Name(cluster=w436, "Pause?"=TRUE) -> (w432:T8)
          }
          frame "Resume" {
            n170 = disable-structure shown="Disabled" {
              frame Disabled {
                n171 = call <vilib>:"Set Busy.vi"() -> ("error out"=w446:errorcluster)  [unwired: 10 in, 1 out]
                n172 = call <vilib>:"Unset Busy.vi"("error in (no error)"=w446) -> ()  [unwired: 10 in, 1 out]
              }
              frame Enabled {
              }
            }
            n173 = Bundle By Name(cluster=w444, "Pause?"=FALSE) -> (w440:T8)
          }
          frame "Stop" {
            w453 = T4 0  # task ID
            n174 = call <vilib>:"Set Busy.vi"() -> ("error out"=w450:errorcluster)  [unwired: 10 in, 1 out]
            n175 = call <vilib>:"Sound Input Stop.vi"("error in (no error)"=w450, "task ID"=w452) -> ("error out"=w448:errorcluster, "task ID out"=w451:T4)  [unwired: 8 in]
            n176 = call <vilib>:"Sound Input Clear.vi"("error in (no error)"=w448, "task ID"=w451) -> ("error out"=w449:errorcluster)  [unwired: 9 in]
            n177 = call <vilib>:"Clear Errors.vi"("error in (no error)"=w449) -> ("error out"=w447:errorcluster)  [unwired: 5 in, 1 out]
            n178 = call <vilib>:"Unset Busy.vi"("error in (no error)"=w447) -> ()  [unwired: 10 in, 1 out]
          }
          frame "Exit" {
            n179 = Unbundle By Name(w462) -> ("data"=w461:refnum<user-event>)
            n180 = Destroy User Event(user event=w461) -> (error out=w460:errorcluster)  [unwired: 1 in]
            n181 = Unregister For Events(event registration refnum=w458, error in=w460) -> (error out=w459:errorcluster)
            n182 = call <vilib>:"Clear Errors.vi"("error in (no error)"=w459) -> ()  [unwired: 5 in, 2 out]
          }
        }
      }
      event Timeout {
        n183 = event-data() -> ()  [unwired: 1 in, 1 out]
        n184 = call-poly <vilib>:"Sound Input Read.vi"("number of samples/ch"=w476, "task ID"=w478) -> ("error out"=w475:errorcluster, "data"=w468:waveform(dbl)[], "task ID out"=w477:T4)  [unwired: 7 in]
        n185 = call <vilib>:"Simple Error Handler.vi"("error in (no error)"=w475) -> ("error out"=w470:errorcluster)  [unwired: 4 in, 4 out]
        n186 = Unbundle By Name(w472) -> ("Pause?"=w471:bool, "data"=w469:refnum<user-event>)
        n187 = case shown="No Error" w470 {
          selector: w470 -> [w483 w491]
          tunnel: w471 -> [w485 _]
          tunnel: [w484 w491] -> w467
          tunnel: w469 -> [w482 _]
          tunnel: w468 -> [w481 _]
          frame No Error {
            n188 = case shown="False" w485 {
              tunnel: [w488 w490] -> w484
              tunnel: w483 -> [w489 w490]
              tunnel: w482 -> [w487 _]
              tunnel: w481 -> [w486 _]
              frame False {
                n189 = Generate User Event(user event=w487, event data cluster=w486, error in=w489) -> (error out=w488:errorcluster)  [unwired: 1 in, 1 out]
              }
              frame True {
              }
            }
          }
          frame Error {
          }
        }
        n190 = Select(t=-1, s=w467, f=w479) -> (s? t:f=w474:i32)
      }
    }
  }
